vi "Gimbal 1.vi"(0 "PITCH 1":fxp<+,32,0>, 2 "frequency (periods/tick)":fxp<+,32,0>, 9 "ROLL1":fxp<+,32,0>, 11 "YAW1":fxp<+,32,0>) -> (4 "DIO 7":bool, 6 "DIO 8":bool, 15 "DIO 9":bool)   [LabVIEW 2015]
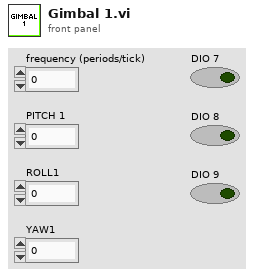
[diagram p1: front panel]
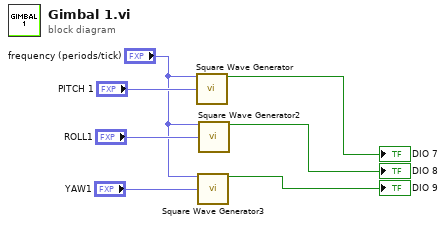
[diagram p0: block diagram]
diagram:
  n1 = call "Square Wave Generator"("frequency (periods/tick)"="frequency (periods/tick)", "duty cycle (periods)"="PITCH 1") -> ("square wave out"=→"DIO 7":bool)  [unwired: 13 in]
  n2 = call "Square Wave Generator3"("frequency (periods/tick)"="frequency (periods/tick)", "duty cycle (periods)"="YAW1") -> ("square wave out"=→"DIO 9":bool)  [unwired: 13 in]
  n3 = call "Square Wave Generator2"("frequency (periods/tick)"="frequency (periods/tick)", "duty cycle (periods)"="ROLL1") -> ("square wave out"=→"DIO 8":bool)  [unwired: 13 in]
